vi "SetDOCoefficients(SubVI).vi"(7 "sn":string, 9 "L":dbl[](array[numeric])) -> (2 "output frame":string)   [LabVIEW 2012]
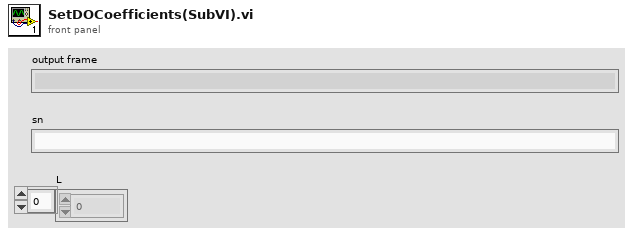
[diagram p1: front panel]
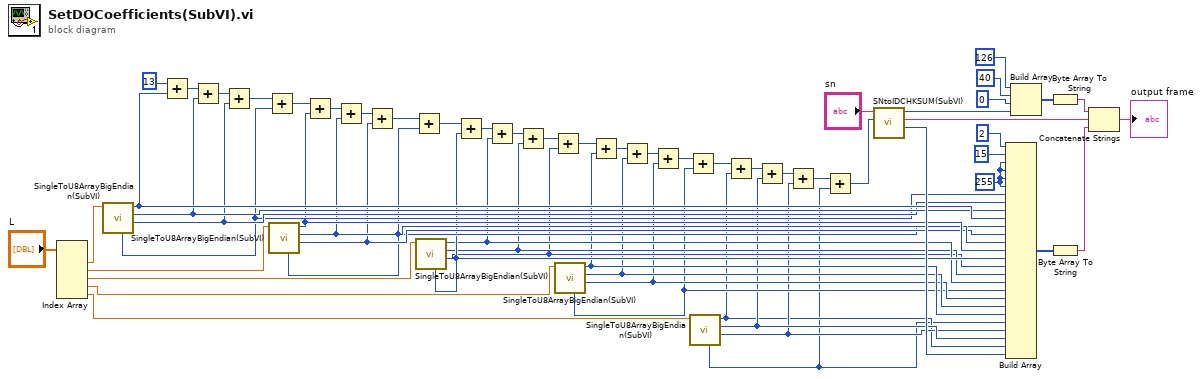
[diagram p0: block diagram]
diagram:
  w60 = u8 255
  n1 = Index Array(array="L") -> (element #1=w5:dbl, element #2=w4:dbl, element #3=w3:dbl, element #4=w2:dbl, element #5=w1:dbl)  [unwired: 5 in]
  n2 = call "SingleToU8ArrayBigEndian(SubVI).vi"("long data"=w5) -> ("third byte"=w42:u8, "send byte"=w45:u8, "first byte"=w46:u8, "forth byte"=w40:u8)  [unwired: 7 in]
  n3 = Add(x=u8 13, y=w46) -> (x+y=w44:u8)
  n4 = Add(x=w44, y=w45) -> (x+y=w43:u8)
  n5 = Add(x=w43, y=w42) -> (x+y=w41:u8)
  n6 = Add(x=w41, y=w40) -> (x+y=w39:u8)
  n7 = call "SingleToU8ArrayBigEndian(SubVI).vi"("long data"=w4) -> ("third byte"=w34:u8, "send byte"=w36:u8, "first byte"=w37:u8, "forth byte"=w32:u8)  [unwired: 7 in]
  n8 = Add(x=w39, y=w37) -> (x+y=w38:u8)
  n9 = Add(x=w38, y=w36) -> (x+y=w35:u8)
  n10 = Add(x=w35, y=w34) -> (x+y=w33:u8)
  n11 = Add(x=w33, y=w32) -> (x+y=w31:u8)
  n12 = call "SingleToU8ArrayBigEndian(SubVI).vi"("long data"=w3) -> ("third byte"=w22:u8, "send byte"=w23:u8, "first byte"=w24:u8, "forth byte"=w25:u8)  [unwired: 7 in]
  n13 = Add(x=w31, y=w25) -> (x+y=w30:u8)
  n14 = Add(x=w30, y=w24) -> (x+y=w29:u8)
  n15 = Add(x=w29, y=w23) -> (x+y=w28:u8)
  n16 = Add(x=w28, y=w22) -> (x+y=w27:u8)
  n17 = call "SingleToU8ArrayBigEndian(SubVI).vi"("long data"=w2) -> ("third byte"=w19:u8, "send byte"=w20:u8, "first byte"=w21:u8, "forth byte"=w18:u8)  [unwired: 7 in]
  n18 = Add(x=w27, y=w21) -> (x+y=w26:u8)
  n19 = Add(x=w26, y=w20) -> (x+y=w17:u8)
  n20 = Add(x=w17, y=w19) -> (x+y=w16:u8)
  n21 = Add(x=w16, y=w18) -> (x+y=w15:u8)
  n22 = call "SingleToU8ArrayBigEndian(SubVI).vi"("long data"=w1) -> ("third byte"=w9:u8, "send byte"=w10:u8, "first byte"=w8:u8, "forth byte"=w7:u8)  [unwired: 7 in]
  n23 = Add(x=w15, y=w8) -> (x+y=w14:u8)
  n24 = Add(x=w14, y=w10) -> (x+y=w13:u8)
  n25 = Add(x=w13, y=w9) -> (x+y=w12:u8)
  n26 = Add(x=w12, y=w7) -> (x+y=w11:u8)
  n27 = call "SNtoIDCHKSUM(SubVI).vi"("fix cheksum"=w11, "input sn"="sn") -> ("output check sum"=w48:u8, "output sn"=w57:string, "output id"=w54:u8)  [unwired: 7 in]
  n28 = Build Array(u8 2, u8 15, w60, w60, w60, w60, w40, w42, w45, w46, w32, w34, w36, w37, w25, w22, w23, w24, w18, w19, w20, w21, w7, w9, w10, w8, w48) -> (w61:u8[])
  n29 = Build Array(u8 126, u8 40, u8 0, w54) -> (w55:u8[])
  n30 = Byte Array To String(unsigned byte array=w55) -> (string=w56:string)
  n31 = Byte Array To String(unsigned byte array=w61) -> (string=w62:string)
  n32 = Concatenate Strings(w56, w57, w62) -> (→"output frame":string)
